vi "GetPubSubListing.vi"(10 "Method":string, 11 "Registered":T1[](array[typedef])) -> (3 "StatusMessage":string)   [LabVIEW 2018]
doc: "Returns status of publisher or subscriber"
uses:
  <userlib>/ROS for LabVIEW Software/ROS/Code/SubVIs/_ROSControl.ctl
  <userlib>/ROS for LabVIEW Software/ROS/Code/SubVIs/_ROSDirection.ctl
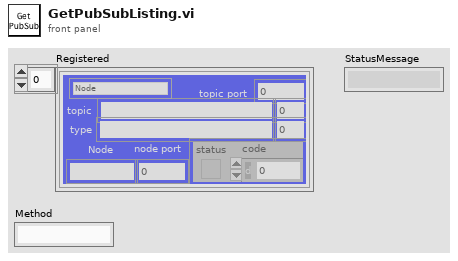
[diagram p1: front panel]
types:
  T1 = typedef "_ROSControl.ctl" = cluster{"topic port":u16, "Node":string, "topic":string, "type":string, "node port":u16, "error ":errorcluster, "Direction":T2, "Update (ms)":u16, "FIFO size":u16}
  T2 = typedef "_ROSDirection.ctl" = enum16{"Node", "Publisher", "Subscriber", "ServiceClient", "ServiceProvider"}
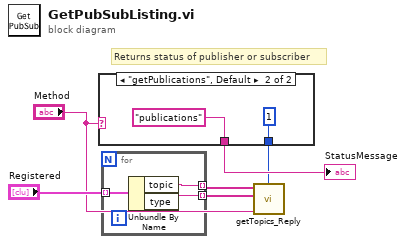
[diagram p0: block diagram]
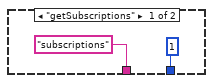
[diagram p2: hidden frame]
diagram:
  # "Returns status of publisher or subscriber"
  n1 = case shown="\"getPublications\", Default" "Method" {
    tunnel: [1 ("Code") 1 ("Code")] -> w5
    tunnel: ["subscriptions" ("StatusMessage") "publications" ("StatusMessage")] -> w6
    frame "getSubscriptions" {
    }
    frame "getPublications", Default {
    }
  }
  "StatusMessage" <- w6
  n2 = for {
    tunnel: "Registered" -> [w13] mode=indexing
    tunnel: [w12] -> w3 mode=indexing
    tunnel: [w11] -> w2 mode=indexing
    n3 = Unbundle By Name(w13) -> ("topic"=w12:string, "type"=w11:string)
  }
  n4 = call <userlib>:"getTopics_Reply.vi"("Code"=w5, "StatusMessage"="Method", "Topic Types"=w2, "Topics"=w3) -> ()  [unwired: 7 in, 1 out]
